vi "RectsEqualEpsilon-lv.vi"(1 "Epsilon":sgl, 2 "B":T1, 3 "A":T1) -> (0 "A == B?":bool)   [LabVIEW 2026, in "SDL3.lvlib" / "Rect.lvlib"]
doc: "<B>LV Implementation</B>\nSince the SDL function is inlined, we can't access in the shared library. So it's a LabVIEW implementation of the feature.\n\n<B>Summary</B>\nDetermine whether two floating point rectangles are equal, within some given epsilon.\n\n<B>Remarks</B>\nRectangles are considered equal if both are not NULL and each of their x, y, width and height are within epsilon of each other. If you don't know what value to use for epsilon, you should call the SDL_RectsEqualFloat function instead."
uses:
  Rect.lvlib
  FRect--cluster.ctl
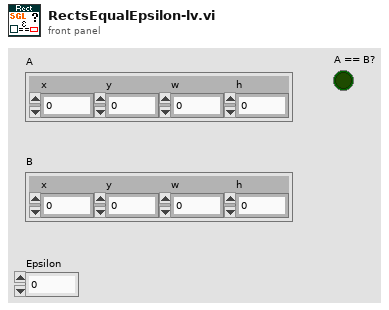
[diagram p1: front panel]
types:
  T1 = typedef "SDL3.lvlib/Rect.lvlib/FRect--cluster.ctl" = cluster{"x":sgl, "y":sgl, "w":sgl, "h":sgl}
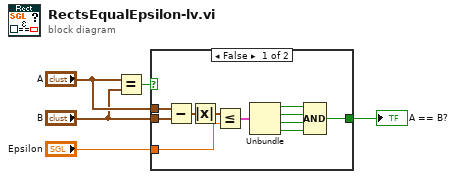
[diagram p0: block diagram]
diagram:
  n1 = Equal?(x="A", y="B") -> (x = y?=w1:bool)
  n2 = case shown="False" w1 {
    selector: w1 -> [_ w17]
    tunnel: "A" -> [w16 _]
    tunnel: "B" -> [w15 _]
    tunnel: "Epsilon" -> [w13 _]
    tunnel: [w7 w17] -> w2
    frame False {
      n3 = Subtract(x=w16, y=w15) -> (x-y=w14:T1)
      n4 = Absolute Value(x=w14) -> (abs(x)=w6:T1)
      n5 = Less Or Equal?(x=w6, y=w13) -> (x <= y?=w12:cluster{"x":bool, "y":bool, "w":bool, "h":bool})
      n6 = Unbundle(w12) -> ("x"=w11:bool, "y"=w9:bool, "w"=w8:bool, "h"=w10:bool)
      n7 = Compound Arithmetic op=AND(w11, w9, w8, w10) -> (w7:bool)
    }
    frame True {
    }
  }
  "A == B?" <- w2
